vi "PololuMacroCommands.vi"(5 "Address":u16=16384 caption="Address [16384=Unadressed]" max=16384, 7 "Port Name (VISA)":refnum<visa-resource-name>, 8 "Error In":errorcluster, 10 "Argument":i32, 11 "Procedure":T1) -> (0 "Error Out":errorcluster, 1 "String Out":string, 2 "Scaled Readback":dbl)   [LabVIEW 2021]
uses:
  TicProcedure.ctl
  PololuCommand.ctl
panel:
  out "GoodReadback":bool
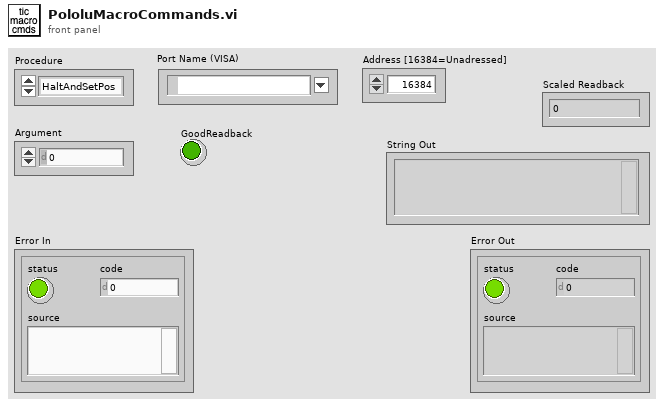
[diagram p1: front panel]
types:
  T1 = typedef "TicProcedure.ctl" = enum16{"HaltAndSetPos", "GetStatus", "GetPosition", "SetTarget", "GetTarget", "Enable", "Disable", "SetCurrent", "GetCurrent", "GetVelocity", "GetUptime", "GetVsupply", "Reset", "Go"}
  T2 = typedef "PololuCommand.ctl" = string
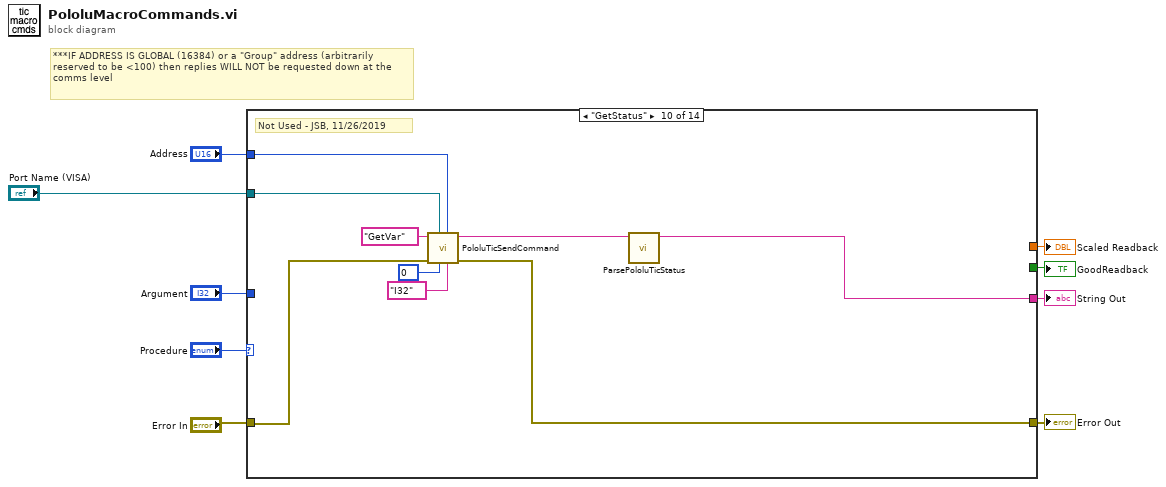
[diagram p0: block diagram]
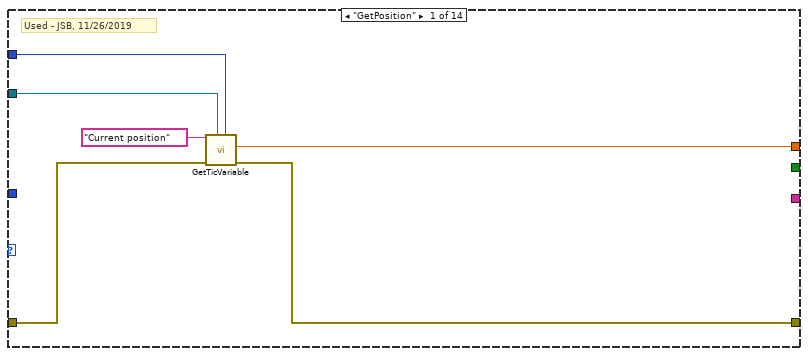
[diagram p2: hidden frame]
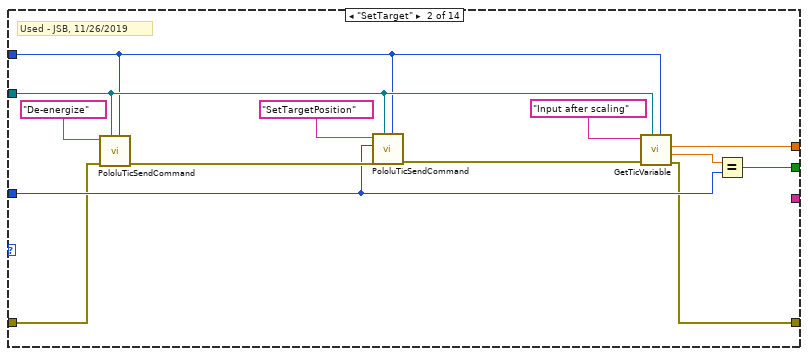
[diagram p3: hidden frame]
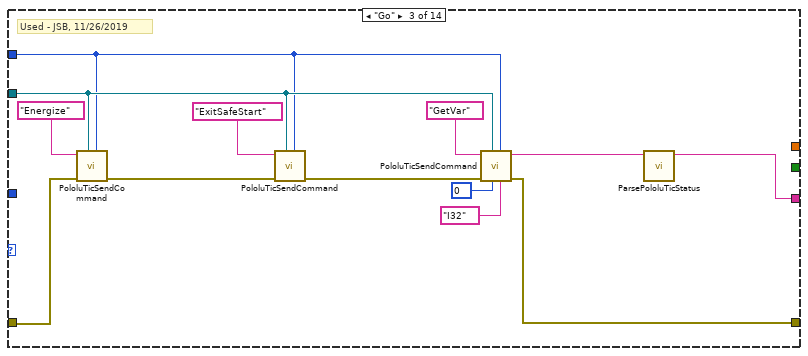
[diagram p4: hidden frame]
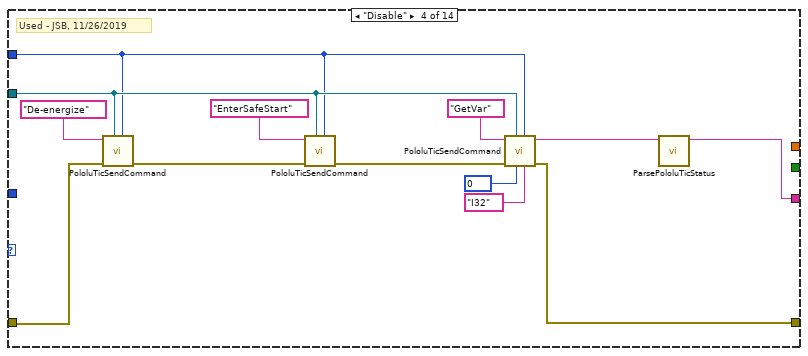
[diagram p5: hidden frame]
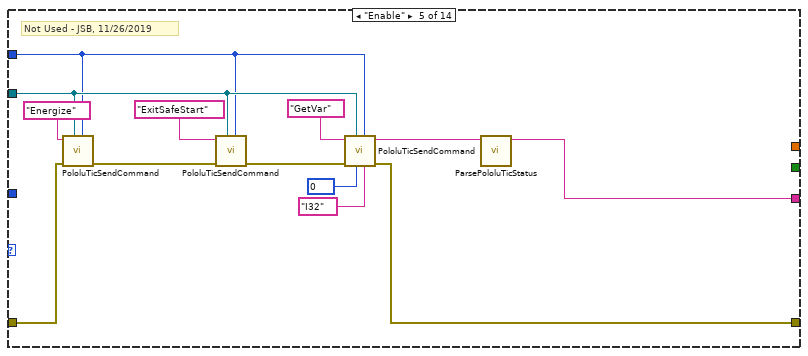
[diagram p6: hidden frame]
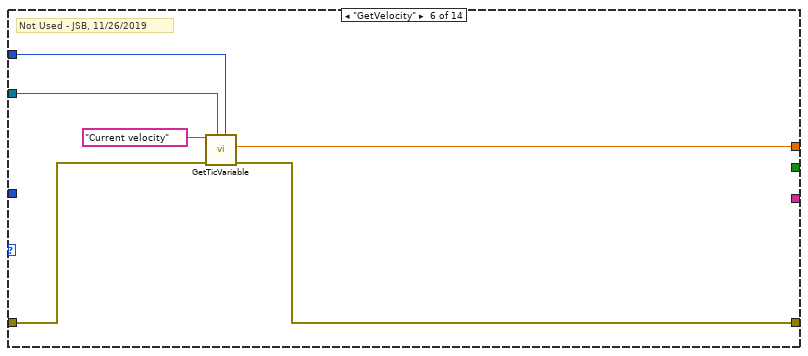
[diagram p7: hidden frame]
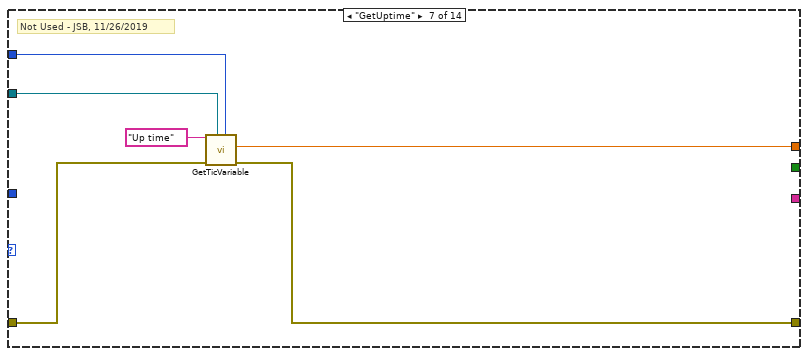
[diagram p8: hidden frame]
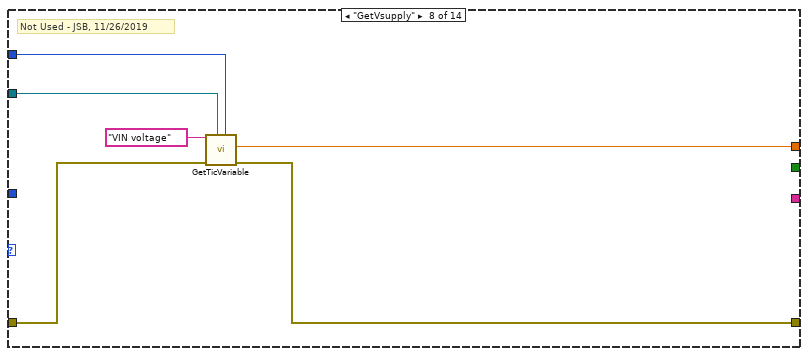
[diagram p9: hidden frame]
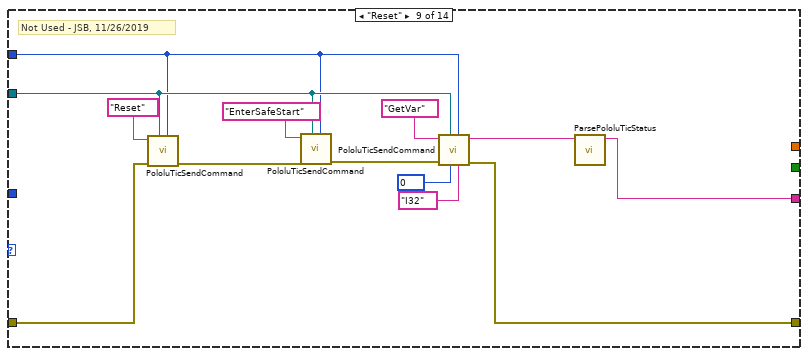
[diagram p10: hidden frame]
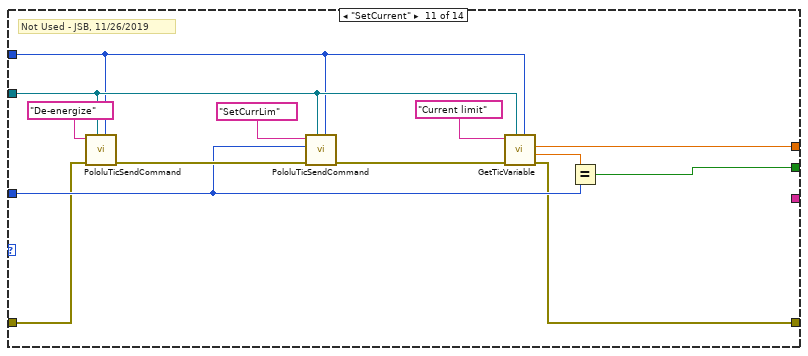
[diagram p11: hidden frame]
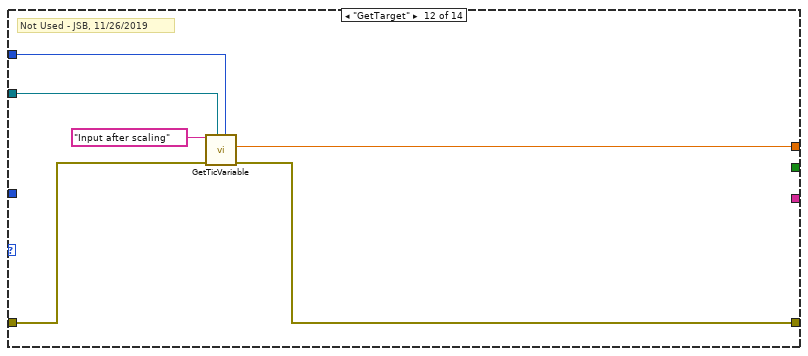
[diagram p12: hidden frame]
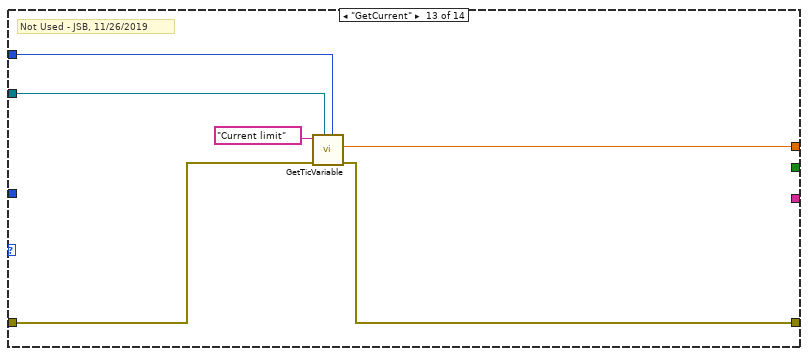
[diagram p13: hidden frame]
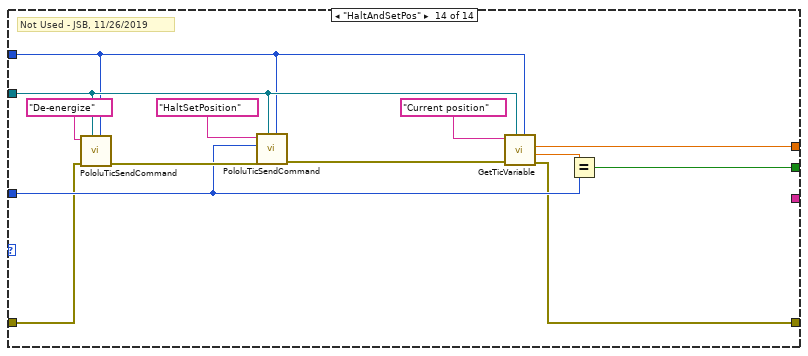
[diagram p14: hidden frame]
diagram:
  # "***IF ADDRESS IS GLOBAL (16384) or a \"Group\" address (arbitrarily reserved to be <100) then replies WILL NOT be requested down at the comms level"
  n1 = case shown="\"GetStatus\"" "Procedure" {
    tunnel: [w10 w17 _ _ _ w68 w74 w80 _ _ w109 w121 w127 w134] -> w8
    tunnel: "Port Name (VISA)" -> [w12 w24 w37 w48 w61 w70 w76 w82 w92 w102 w116 w123 w132 w141]
    tunnel: "Argument" -> [_ w23 _ _ _ _ _ _ _ _ w115 _ _ w140]
    tunnel: [_ w22 _ _ _ _ _ _ _ _ w114 _ _ w139] -> w6
    tunnel: [_ _ w35 w47 w60 _ _ _ w90 w107 _ _ _ _] -> w5
    tunnel: "Address" -> [w11 w21 w34 w45 w56 w69 w75 w81 w89 w105 w113 w122 w131 w138]
    tunnel: "Error In" -> [w13 w20 w33 w44 w58 w71 w77 w83 w88 w103 w112 w124 w130 w137]
    tunnel: [w14 w19 w32 w43 w57 w72 w78 w84 w87 w101 w111 w125 w129 w136] -> w2
    frame "GetPosition" {
      # "Used - JSB, 11/26/2019"
      n2 = call "GetTicVariable.vi"("Address [16384=Unadressed/Global]"=w11, "Port Name (VISA)"=w12, "errorIn"=w13, "Variable"="Current position") -> ("errorOut"=w14:errorcluster, "Value"=w10:dbl)  [unwired: 4 in, 2 out]
    }
    frame "SetTarget" {
      # "Used - JSB, 11/26/2019"
      n3 = call "PololuTicSendCommand.vi"("Address"=w21, "Port Name"=w24, "errorIn"=w20, "PololuCommand"=T2 "De-energize") -> ("errorOut"=w25:errorcluster)  [unwired: 4 in, 3 out]
      n4 = call "PololuTicSendCommand.vi"("Address"=w21, "Port Name"=w24, "errorIn"=w25, "Argument"=w23, "PololuCommand"=T2 "SetTargetPosition") -> ("errorOut"=w27:errorcluster)  [unwired: 3 in, 3 out]
      n5 = call "GetTicVariable.vi"("Address [16384=Unadressed/Global]"=w21, "Port Name (VISA)"=w24, "errorIn"=w27, "Variable"="Input after scaling") -> ("errorOut"=w19:errorcluster, "RawValueRead"=w16:dbl, "Value"=w17:dbl)  [unwired: 4 in, 1 out]
      n6 = Equal?(x=w16, y=w23) -> (x = y?=w22:bool)
    }
    frame "Go" {
      # "Used - JSB, 11/26/2019"
      n7 = call "PololuTicSendCommand.vi"("Address"=w34, "Port Name"=w37, "errorIn"=w33, "PololuCommand"=T2 "Energize") -> ("errorOut"=w38:errorcluster)  [unwired: 4 in, 3 out]
      n8 = call "PololuTicSendCommand.vi"("Address"=w34, "Port Name"=w37, "errorIn"=w38, "PololuCommand"=T2 "ExitSafeStart") -> ("errorOut"=w40:errorcluster)  [unwired: 4 in, 3 out]
      n9 = call "PololuTicSendCommand.vi"("Type"="I32", "Address"=w34, "Register"=u8 0, "Port Name"=w37, "errorIn"=w40, "PololuCommand"=T2 "GetVar") -> ("errorOut"=w32:errorcluster, "Response"=w36:string)  [unwired: 2 in, 2 out]
      n10 = call "ParsePololuTicStatus.vi"("BytesIn"=w36) -> ("String"=w35:string)  [unwired: 10 in]
    }
    frame "Disable" {
      # "Used - JSB, 11/26/2019"
      n11 = call "PololuTicSendCommand.vi"("Address"=w45, "Port Name"=w48, "errorIn"=w44, "PololuCommand"=T2 "De-energize") -> ("errorOut"=w49:errorcluster)  [unwired: 4 in, 3 out]
      n12 = call "PololuTicSendCommand.vi"("Address"=w45, "Port Name"=w48, "errorIn"=w49, "PololuCommand"=T2 "EnterSafeStart") -> ("errorOut"=w52:errorcluster)  [unwired: 4 in, 3 out]
      n13 = call "PololuTicSendCommand.vi"("Type"="I32", "Address"=w45, "Register"=u8 0, "Port Name"=w48, "errorIn"=w52, "PololuCommand"=T2 "GetVar") -> ("errorOut"=w43:errorcluster, "Response"=w46:string)  [unwired: 2 in, 2 out]
      n14 = call "ParsePololuTicStatus.vi"("BytesIn"=w46) -> ("String"=w47:string)  [unwired: 10 in]
    }
    frame "Enable" {
      # "Not Used - JSB, 11/26/2019"
      n15 = call "PololuTicSendCommand.vi"("Address"=w56, "Port Name"=w61, "errorIn"=w58, "PololuCommand"=T2 "Energize") -> ("errorOut"=w62:errorcluster)  [unwired: 4 in, 3 out]
      n16 = call "PololuTicSendCommand.vi"("Address"=w56, "Port Name"=w61, "errorIn"=w62, "PololuCommand"=T2 "ExitSafeStart") -> ("errorOut"=w65:errorcluster)  [unwired: 4 in, 3 out]
      n17 = call "PololuTicSendCommand.vi"("Type"="I32", "Address"=w56, "Register"=u8 0, "Port Name"=w61, "errorIn"=w65, "PololuCommand"=T2 "GetVar") -> ("errorOut"=w57:errorcluster, "Response"=w59:string)  [unwired: 2 in, 2 out]
      n18 = call "ParsePololuTicStatus.vi"("BytesIn"=w59) -> ("String"=w60:string)  [unwired: 10 in]
    }
    frame "GetVelocity" {
      # "Not Used - JSB, 11/26/2019"
      n19 = call "GetTicVariable.vi"("Address [16384=Unadressed/Global]"=w69, "Port Name (VISA)"=w70, "errorIn"=w71, "Variable"="Current velocity") -> ("errorOut"=w72:errorcluster, "Value"=w68:dbl)  [unwired: 4 in, 2 out]
    }
    frame "GetUptime" {
      # "Not Used - JSB, 11/26/2019"
      n20 = call "GetTicVariable.vi"("Address [16384=Unadressed/Global]"=w75, "Port Name (VISA)"=w76, "errorIn"=w77, "Variable"="Up time") -> ("errorOut"=w78:errorcluster, "Value"=w74:dbl)  [unwired: 4 in, 2 out]
    }
    frame "GetVsupply" {
      # "Not Used - JSB, 11/26/2019"
      n21 = call "GetTicVariable.vi"("Address [16384=Unadressed/Global]"=w81, "Port Name (VISA)"=w82, "errorIn"=w83, "Variable"="VIN voltage") -> ("errorOut"=w84:errorcluster, "Value"=w80:dbl)  [unwired: 4 in, 2 out]
    }
    frame "Reset" {
      # "Not Used - JSB, 11/26/2019"
      n22 = call "PololuTicSendCommand.vi"("Address"=w89, "Port Name"=w92, "errorIn"=w88, "PololuCommand"=T2 "Reset") -> ("errorOut"=w93:errorcluster)  [unwired: 4 in, 3 out]
      n23 = call "PololuTicSendCommand.vi"("Address"=w89, "Port Name"=w92, "errorIn"=w93, "PololuCommand"=T2 "EnterSafeStart") -> ("errorOut"=w96:errorcluster)  [unwired: 4 in, 3 out]
      n24 = call "PololuTicSendCommand.vi"("Type"="I32", "Address"=w89, "Register"=u8 0, "Port Name"=w92, "errorIn"=w96, "PololuCommand"=T2 "GetVar") -> ("errorOut"=w87:errorcluster, "Response"=w91:string)  [unwired: 2 in, 2 out]
      n25 = call "ParsePololuTicStatus.vi"("BytesIn"=w91) -> ("String"=w90:string)  [unwired: 10 in]
    }
    frame "GetStatus" {
      # "Not Used - JSB, 11/26/2019"
      n26 = call "PololuTicSendCommand.vi"("Type"="I32", "Address"=w105, "Register"=u8 0, "Port Name"=w102, "errorIn"=w103, "PololuCommand"=T2 "GetVar") -> ("errorOut"=w101:errorcluster, "Response"=w104:string)  [unwired: 2 in, 2 out]
      n27 = call "ParsePololuTicStatus.vi"("BytesIn"=w104) -> ("String"=w107:string)  [unwired: 10 in]
    }
    frame "SetCurrent" {
      # "Not Used - JSB, 11/26/2019"
      n28 = call "PololuTicSendCommand.vi"("Address"=w113, "Port Name"=w116, "errorIn"=w112, "PololuCommand"=T2 "De-energize") -> ("errorOut"=w117:errorcluster)  [unwired: 4 in, 3 out]
      n29 = call "PololuTicSendCommand.vi"("Address"=w113, "Port Name"=w116, "errorIn"=w117, "Argument"=w115, "PololuCommand"=T2 "SetCurrLim") -> ("errorOut"=w119:errorcluster)  [unwired: 3 in, 3 out]
      n30 = call "GetTicVariable.vi"("Address [16384=Unadressed/Global]"=w113, "Port Name (VISA)"=w116, "errorIn"=w119, "Variable"="Current limit") -> ("errorOut"=w111:errorcluster, "RawValueRead"=w108:dbl, "Value"=w109:dbl)  [unwired: 4 in, 1 out]
      n31 = Equal?(x=w108, y=w115) -> (x = y?=w114:bool)
    }
    frame "GetTarget" {
      # "Not Used - JSB, 11/26/2019"
      n32 = call "GetTicVariable.vi"("Address [16384=Unadressed/Global]"=w122, "Port Name (VISA)"=w123, "errorIn"=w124, "Variable"="Input after scaling") -> ("errorOut"=w125:errorcluster, "Value"=w121:dbl)  [unwired: 4 in, 2 out]
    }
    frame "GetCurrent" {
      # "Not Used - JSB, 11/26/2019"
      n33 = call "GetTicVariable.vi"("Address [16384=Unadressed/Global]"=w131, "Port Name (VISA)"=w132, "errorIn"=w130, "Variable"="Current limit") -> ("errorOut"=w129:errorcluster, "Value"=w127:dbl)  [unwired: 4 in, 2 out]
    }
    frame "HaltAndSetPos" {
      # "Not Used - JSB, 11/26/2019"
      n34 = call "PololuTicSendCommand.vi"("Address"=w138, "Port Name"=w141, "errorIn"=w137, "PololuCommand"=T2 "De-energize") -> ("errorOut"=w142:errorcluster)  [unwired: 4 in, 3 out]
      n35 = call "PololuTicSendCommand.vi"("Address"=w138, "Port Name"=w141, "errorIn"=w142, "Argument"=w140, "PololuCommand"=T2 "HaltSetPosition") -> ("errorOut"=w144:errorcluster)  [unwired: 3 in, 3 out]
      n36 = call "GetTicVariable.vi"("Address [16384=Unadressed/Global]"=w138, "Port Name (VISA)"=w141, "errorIn"=w144, "Variable"="Current position") -> ("errorOut"=w136:errorcluster, "RawValueRead"=w133:dbl, "Value"=w134:dbl)  [unwired: 4 in, 1 out]
      n37 = Equal?(x=w133, y=w140) -> (x = y?=w139:bool)
    }
  }
  "Scaled Readback" <- w8
  "GoodReadback" <- w6
  "String Out" <- w5
  "Error Out" <- w2
